vi "Running Wrapper.vi"(8 "error in (no error)":errorcluster, 11 "CIFPlugin in":refnum<class "Template_Plugin.lvclass">) -> (0 "error out":errorcluster, 2 "Destroy":bool, 3 "CIFPlugin out":refnum<class "Template_Plugin.lvclass">)   [LabVIEW 2021, in "Template_Plugin.lvclass"]
doc: "Wrapper around the Core Running VI. This wrapper will handle selection of timed loop with priorities or execution without a timed loop. \n\nIf the VI is compiled to run on LinuxRT it will check if timed loop is supported (RT compiled PPLs can run on desktop but timed loop is not supported and conditional compile will not check after PPL is compiled). If the timed loop is supported it will check if the priority is a positive value. If positive it will run in timed loop and set priority. A negative value will indicate configuration to not used timed loop."
uses:
  Template_Plugin.lvclass
  C:/Program Files/National Instruments/LabVIEW 2021/vi.lib/CIF Foundation/CIF Core/CIFCore/Class/CIFCorePlugin.lvclass
  <vilib>/CIF Foundation/CIF Core/CIFCore/Class/CIFCorePlugin.lvclass/CIFCorePlugin.ctl
  <vilib>/CIF Foundation/CIF Utilities/Statistics/I64/Stats_I64_CIF_U.lvclass/Stats_I64_CIF_U.ctl
  Template_Plugin.lvclass/Template_Plugin.ctl
  <vilib>/CIF Foundation/CIF Core/Channels/CIFChannelMng/CIFChannelMng.lvclass/CIFChannelMng.ctl
  <vilib>/CIF Foundation/CIF Channels Core/CIFChannels/CIFChannels.lvclass/CIFChannels.ctl
  <vilib>/CIF Foundation/CIF Core/CIFCore/Class/SubVIs/Running State Logic.vi
  Execution/Execute.vi
  Execution/Housekeeping.vi
  <vilib>/CIF Foundation/CIF Core/CIFCore/Class/SubVIs/OOB/Send Core OOB TX.vi
  <vilib>/CIF Foundation/CIF Core/CIFCore/Class/Accessors/Read Energized State.vi
  <vilib>/CIF Foundation/CIF Core/CIFCore/Class/SubVIs/Start Running.vi
  Execution/Logic.vi
  <vilib>/CIF Foundation/CIF Core/CIFCore/Class/Accessors/Write Energized State.vi
  <vilib>/CIF Foundation/CIF Core/CIFCore/Class/SubVIs/Timing/Sleep.vi
  <vilib>/CIF Foundation/CIF Core/CIFCore/Class/Benchmarking/Benchmark Running.vi
  <vilib>/CIF Foundation/CIF Core/CIFCore/Class/SubVIs/OOB/Read Core OOB RX.vi
  OOB Comm/Read Comm to Main.vi
  OOB Comm/Send Cyclic to gRPC.vi
  <vilib>/CIF Foundation/CIF Core/CIFCore/Class/Benchmarking/Benchmark Housekeeping.vi
  <vilib>/CIF Foundation/CIF Core/CIFCore/Class/SubVIs/OOB/Update Status from Benchmarks.vi
  <vilib>/CIF Foundation/CIF Core/Channels/CIFChannelMng/Core/Send Channel List Update.vi
  <vilib>/CIF Foundation/CIF Core/CIFCore/Class/SubVIs/OOB/Send Core OOB TX.vi/074d8088-3ad4-4fdc-9542-b009f1b06b72.vi
  <vilib>/CIF Foundation/CIF Utilities/Time/System Time/Sleep Until Future Time.vi
  <vilib>/CIF Foundation/CIF Utilities/Time/System Time/Get System Time.vi
  <vilib>/CIF Foundation/CIF Core/CIFCore/Class/Accessors/Timestamps/Write Execute TS.vi
  <vilib>/Utility/error.llb/Clear Errors.vi
  <vilib>/CIF Foundation/CIF Core/CIFCore/Class/Accessors/Read Sleep Limits (ns).vi
  <vilib>/CIF Foundation/CIF Core/CIFCore/Class/Accessors/Timestamps/Write Target Wake TS.vi
  <vilib>/CIF Foundation/CIF Core/CIFCore/Class/Accessors/Read Plugin Name.vi
  <vilib>/CIF Foundation/CIF Core/CIFCore/Common/Utilities/Add Error.vi
  <vilib>/CIF Foundation/CIF Core/CIFCore/Class/Accessors/Timestamps/Read Running TS.vi
  <vilib>/CIF Foundation/CIF Core/CIFCore/Class/Accessors/Timestamps/Write Sleep TS.vi
  <vilib>/CIF Foundation/CIF Core/CIFCore/Class/Benchmarking/Reset Delay.vi
  <vilib>/CIF Foundation/CIF Core/CIFCore/Class/Accessors/Read Timing Override.vi
  <vilib>/CIF Foundation/CIF Core/CIFCore/Class/Accessors/Read Common Config.vi
  <vilib>/CIF Foundation/CIF Core/CIFCore/Class/Benchmarking/Benchmark Execute.vi
  <vilib>/CIF Foundation/CIF Core/CIFCore/Class/Accessors/Timestamps/Write Housekeeping TS.vi
  <vilib>/CIF Foundation/CIF Core/CIFCore/Class/SubVIs/Refresh Stats.vi
  <vilib>/CIF Foundation/CIF Core/CIFCore/Class/SubVIs/OOB/Receive/Read Clock Map.vi
  <vilib>/CIF Foundation/CIF Core/CIFCore/Class/SubVIs/OOB/Receive/Read Connections.vi
  <vilib>/CIF Foundation/CIF Core/Channels/CIFChannelMng/SubVIs/Connect Channel.vi
  <vilib>/CIF Foundation/CIF Core/CIFCore/Class/SubVIs/OOB/Receive/Read Forces.vi
  <vilib>/CIF Foundation/CIF Core/Channels/CIFChannelMng/SubVIs/Force Channel.vi
  <vilib>/CIF Foundation/CIF Core/Channels/CIFChannelMng/SubVIs/Add FIFO Publisher.vi
  <vilib>/CIF Foundation/CIF Core/CIFCore/Class/SubVIs/OOB/Receive/Read Publisher Instance.vi
  <vilib>/CIF Foundation/CIF Core/Channels/CIFChannelMng/Core/Send Publisher Instance Return.vi
  <vilib>/CIF Foundation/CIF Core/Channels/CIFChannelMng/SubVIs/Remove FIFO Publisher.vi
  <vilib>/CIF Foundation/CIF Core/CIFCore/Class/SubVIs/OOB/Read Core OOB RX.vi/a31a91a9-4107-4750-8e0d-44486e9a3a34.vi
  OOB Comm/Read Comm to Main.vi/4efb0375-f1de-4191-b03f-44d34e6646cb.vi
  OOB Comm/Read Comm to Main.vi/525c214c-2a6b-4e7b-b3ce-0ad96b412d2f.vi
  OOB Comm/Send Cyclic to gRPC.vi/0c0f428d-7269-422d-ba27-f9d6fa7232ec.vi
  <vilib>/CIF Foundation/CIF Core/CIFCore/Class/Accessors/Read Refresh.vi
  <vilib>/CIF Foundation/CIF Utilities/Statistics/I64/X1 minus X0.vi
  <vilib>/CIF Foundation/CIF Core/CIFCore/Class/Accessors/Timestamps/Read Housekeeping TS.vi
  <vilib>/CIF Foundation/CIF Utilities/Statistics/I64/Get Stats.vi
  <vilib>/CIF Foundation/CIF Core/Channels/CIFChannelMng/Core/Send Channel List Update.vi/463ebf4c-8748-40f9-8ad3-9e61c16a01a6.vi
  <vilib>/CIF Foundation/CIF CIPC/SubVIs/Check Error.vi
  <vilib>/CIF Foundation/CIF CIPC/SubVIs/Notify Of New Write.vi
  <vilib>/CIF Foundation/CIF CIPC/SubVIs/Get dll Path.vi
  <vilib>/CIF Foundation/CIF CIPC/SubVIs/Get Element Write Position.vi
  <vilib>/CIF Foundation/CIF Utilities/Time/SubVIs/Add Error.vi
  <vilib>/CIF Foundation/CIF Utilities/Time/System Time/LabVIEW Time to TAI Time.vi
  <vilib>/CIF Foundation/CIF Utilities/Errors/Append Error Location.vi
  <vilib>/CIF Foundation/CIF Utilities/Statistics/I64/Cyclic.vi
  <vilib>/CIF Foundation/CIF Core/CIFCore/Class/Accessors/Timestamps/Read Execute TS.vi
  <vilib>/CIF Foundation/CIF Core/CIFCore/Class/Accessors/Timestamps/Read Sleep TS.vi
  <vilib>/CIF Foundation/CIF Core/CIFCore/Class/Accessors/Timestamps/Read Target Wake TS.vi
  <vilib>/CIF Foundation/CIF Core/Channels/CIFChannelMng/Utilities/Get Channel Index by Name.vi
  <vilib>/CIF Foundation/CIF Channels Core/CIFChannels/Accessors/Read Channel State.vi
  <vilib>/CIF Foundation/CIF Channels Core/CIFChannels/Accessors/Read Tag Forced.vi
  <vilib>/CIF Foundation/CIF Core/Channels/CIFChannelMng/SubVIs/Add Error Channel Manager.vi
  <vilib>/CIF Foundation/CIF Core/Channels/CIFChannelMng/Core/Send Publisher Instance Return.vi/9db40550-ae0b-4108-a32d-02e81b824dbe.vi
  <vilib>/CIF Foundation/CIF Core/Channels/CIFChannelMng/SubVIs/Get Original FIFO Channel Name.vi
  <vilib>/CIF Foundation/CIF CIPC/SubVIs/Wait For N Elements Available.vi
  <vilib>/CIF Foundation/CIF CIPC/SubVIs/Get Element Read Position.vi
  <vilib>/CIF Foundation/CIF CIPC/SubVIs/Set Element Read Position.vi
  <vilib>/CIF Foundation/CIF Utilities/Statistics/I64/X1 minus X0.vi/dfabcf33-0dbc-4041-80a5-3dc0c86d2989.vi
  <vilib>/CIF Foundation/CIF Utilities/Statistics/I64/Cyclic.vi/dfabcf33-0dbc-4041-80a5-3dc0c86d2989.vi
  <vilib>/CIF Foundation/CIF Channels Core/ChannelCommon/Utilities/Add Error.vi
  <vilib>/CIF Foundation/CIF Utilities/Statistics/I64/X1 minus X0.vi/dfabcf33-0dbc-4041-80a5-3dc0c86d2989.vi/9eb60a9a-770f-4d2d-8b3f-8465c267ecc9.vi
  <vilib>/CIF Foundation/CIF Utilities/Statistics/I64/Cyclic.vi/dfabcf33-0dbc-4041-80a5-3dc0c86d2989.vi/9eb60a9a-770f-4d2d-8b3f-8465c267ecc9.vi
  <vilib>/CIF Foundation/CIF Core/CIFCore/Class/Logs/Log Run.vi
  <vilib>/CIF Foundation/CIF CIPC/SubVIs/Get Element Info Variant.vi
  <vilib>/Utility/error.llb/Trim Whitespace.vi
  <vilib>/Utility/error.llb/Error Cluster From Error Code.vi
  <vilib>/CIF Foundation/CIF Channels Core/CIFChannels/Core/Set Force.vi
  <vilib>/CIF Foundation/CIF Core/CIFCore/Class/Top Level/Core Handle Error.vi
  <vilib>/CIF Foundation/CIF Core/CIFCore/Class/CIFCorePlugin.lvclass
  <vilib>/CIF Foundation/CIF Channels Core/CIFChannels/CIFChannels.lvclass
  <vilib>/Platform/TimedLoop/XDataNode/wakeup.ctl
  <vilib>/Platform/TimedLoop/XDataNode/XDNodeRunTimeDep.lvlib
  <vilib>/Platform/TimedLoop/XDataNode/nitl_modes.ctl
  <vilib>/Platform/TimedLoop/XDataNode/timing_clust.ctl
  <vilib>/Platform/TimedLoop/XDataNode/XDataNode.xnode
  D:/dev/Plugins/Template/src/Source/CIF/Plugin Generator/Template/Class/Template_Plugin.lvclass
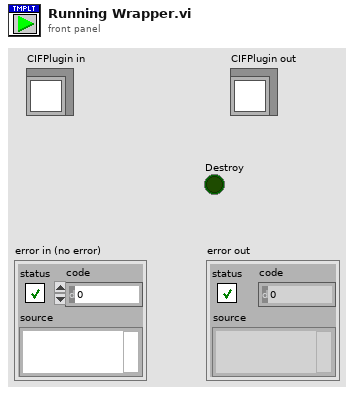
[diagram p1: front panel]
types:
  T1 = typedef "XDNodeRunTimeDep.lvlib/timing_clust.ctl" = cluster{"Expected End [f-1]":u64, "Actual End [f-1]":u64, "Finished Late? [f-1]":bool, "Expected End [i-1]":u64, "Actual End [i-1]":u64, "Finished Late? [i-1]":bool, "Expected Start [i]":u64, "Actual Start [i]":u64, "Expected Start [f]":u64, "Actual Start [f]":u64, "Source Name":string, "Structure Name":string, "Period":i64, "Deadline":i64, "Offset":i64, "Start":i64, "Priority":i32, "Timeout":i32, "Mode":T2, "Wakeup Reason":T3, "Error":errorcluster, "Source Type":string, "Secondary Source Type":string, "Global End Time":u64, "Global Start Time":u64, "Frame Duration":u64, "Iteration Duration":u64, "Assigned CPU":i32, "I/O Scan Engine Mode":u32}
  T2 = typedef "XDNodeRunTimeDep.lvlib/nitl_modes.ctl" = enum32{"No Change", "Process missed periods, maintain original phase", "Discard missed periods, maintain original phase", "Process missed periods, ignore original phase", "Discard missed periods, ignore original phase"}
  T3 = typedef "XDNodeRunTimeDep.lvlib/wakeup.ctl" = enum32{"Normal", "Aborted", "Asynchronous wakeup", "Timing source error", "Timed loop error", "Timeout"}
  T4 = typedef "CIFCorePlugin.lvclass/Running Internal Data.ctl" = cluster{"Refresh":bool, "Iterations":i64, "Housekeep only":bool, "Configured period (ns)":i64, "Update channel OOB":bool, "Configuration Change":bool, "Disable Auto Benchmark":bool, "gRPC Loop":bool, "Timed Loop Supported":bool}
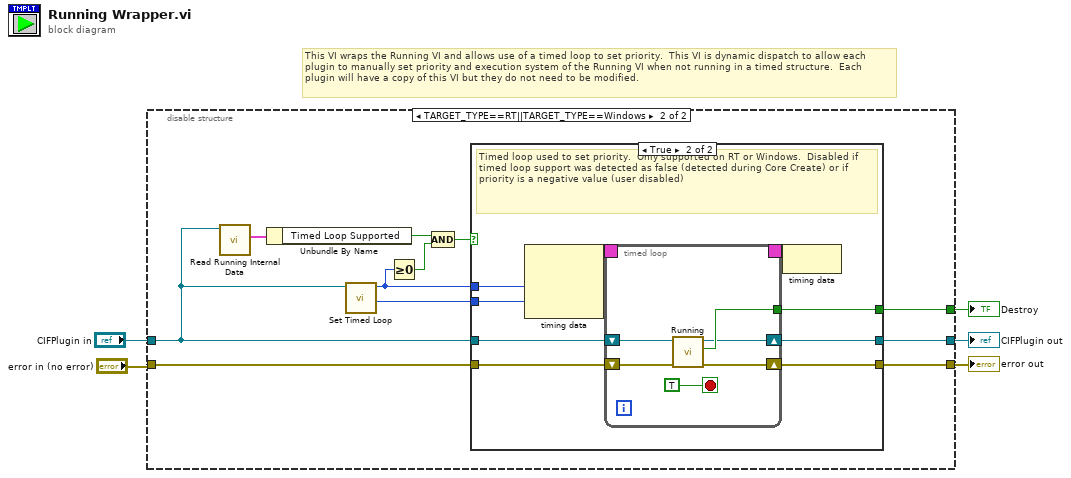
[diagram p0: block diagram]
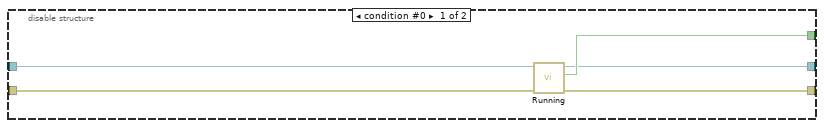
[diagram p2: hidden frame]
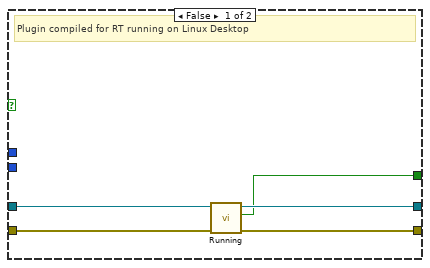
[diagram p3: hidden frame]
diagram:
  # "This VI wraps the Running VI and allows use of a timed loop to set priority.  This VI is dynamic dispatch to allow each plugin to manually set priority and execution system of the Running VI when not running in a timed structure.  Each plugin will have a copy of this VI but they do not need to be modified."
  n1 = disable-structure shown="TARGET_TYPE==RT||TARGET_TYPE==Windows" {
    disable-tunnel: "CIFPlugin in" -> [w6 w12]
    disable-tunnel: "error in (no error)" -> [w10 w21]
    disable-tunnel: [w8 w20] -> w3
    disable-tunnel: [w7 w19] -> w1
    disable-tunnel: [w9 w18] -> w4
    frame condition #0 {
      n2 = call "Running.vi"("error in (no error)"=w10, "CIFPlugin in"=w6) -> ("error out"=w9:errorcluster, "Destroy"=w8:bool, "CIFPlugin out"=w7:refnum<class "Template_Plugin.lvclass">)  [unwired: 7 in]
    }
    frame condition #1 (active) {
      n3 = call <vilib>:"Read Running Internal Data.vi"("CIFCorePlugin in"=w12) -> ("Running Internal Data"=w11:T4)  [unwired: 8 in, 2 out]
      n4 = Unbundle By Name(w11) -> ("Timed Loop Supported"=w15:bool)
      n5 = call <vilib>:"Set Timed Loop.vi"("CIFCorePlugin in"=w12) -> ("Processor"=w17:i32, "Priority"=w16:i32)  [unwired: 9 in]
      n6 = Greater Or Equal To 0?(x=w16) -> (x >= 0?=w14:bool)
      n7 = Compound Arithmetic op=AND(w15, w14) -> (w13:bool)
      n8 = case shown="True" w13 {
        tunnel: w21 -> [w25 w33]
        tunnel: [w22 w32] -> w20
        tunnel: [w24 w31] -> w19
        tunnel: [w23 w30] -> w18
        tunnel: w12 -> [w26 w29]
        tunnel: w16 -> [_ w28]
        tunnel: w17 -> [_ w27]
        frame False {
          # "Plugin compiled for RT running on Linux Desktop"
          n9 = call "Running.vi"("error in (no error)"=w25, "CIFPlugin in"=w26) -> ("error out"=w23:errorcluster, "Destroy"=w22:bool, "CIFPlugin out"=w24:refnum<class "Template_Plugin.lvclass">)  [unwired: 7 in]
        }
        frame True {
          # "Timed loop used to set priority.  Only supported on RT or Windows.  Disabled if timed loop support was detected as false (detected during Core Create) or if priority is a negative value (user disabled)"
          n10 = node-c288(w28, w27) -> (w35:T1)  [unwired: 1 in]
          n11 = timed-loop {
            timing: w35 -> [_]
            timing-out: [_] -> w34
            shift-right: [w36] -> w31
            shift-left: w29 -> [w40]
            shift-right: [w38] -> w30
            shift-left: w33 -> [w39]
            tunnel: [w37] -> w32
            stop <- TRUE stop-if-true
            n12 = call "Running.vi"("error in (no error)"=w39, "CIFPlugin in"=w40) -> ("error out"=w38:errorcluster, "Destroy"=w37:bool, "CIFPlugin out"=w36:refnum<class "Template_Plugin.lvclass">)  [unwired: 7 in]
          }
          n13 = node-c288(w34) -> ()
        }
      }
    }
  }
  "error out" <- w4
  "Destroy" <- w3
  "CIFPlugin out" <- w1
